vi "empty_string_values.vi"(11 "string refs":refnum<vi>[](array[refnum])) -> ()   [LabVIEW 2013]
panel:
  in  "Rino status control":T1={"Navigation controls"={"full path tree"=refnum, "folder content tree"=refnum, "next page"=refnum, "previous page"=refnum, "refresh file list"=refnum, "delete"=refnum, "page indicator string"=refnum}, "New Folder controls"={"next folder"=refnum, "name"="", "tags"="", "notes"="", "metadata array"=[]}, "Upload File controls"={"upoad file"=refnum, "name"="", "tags"="", "notes"="", "metadata array"=[], "Store data locally"=TRUE, "Store metadata locally"=FALSE, "Path Refnum"=refnum}, "Metadata management controls"={"get metadata"=refnum, "update metadata"=refnum, "name"=refnum, "tags"=refnum, "notes"=refnum, "metadata tree"=refnum}, "Status indicators"={"error"=refnum, "active item"=refnum, "last action"=refnum, "http header"=refnum, "http body"=refnum}, "Move file controls"={"source item"=refnum, "destination item"=refnum, "set source"=refnum, "set destination"=refnum, "move"=refnum}} {"Upload File controls"."metadata array"."Data type" items=["Numeric", "String", "1D array of strings", "1D array of doubles", "Data JSON string", "<null>"]; "New Folder controls"."metadata array"."Data type" items=["Numeric", "String", "1D array of strings", "1D array of doubles", "Data JSON string", "<null>"]}
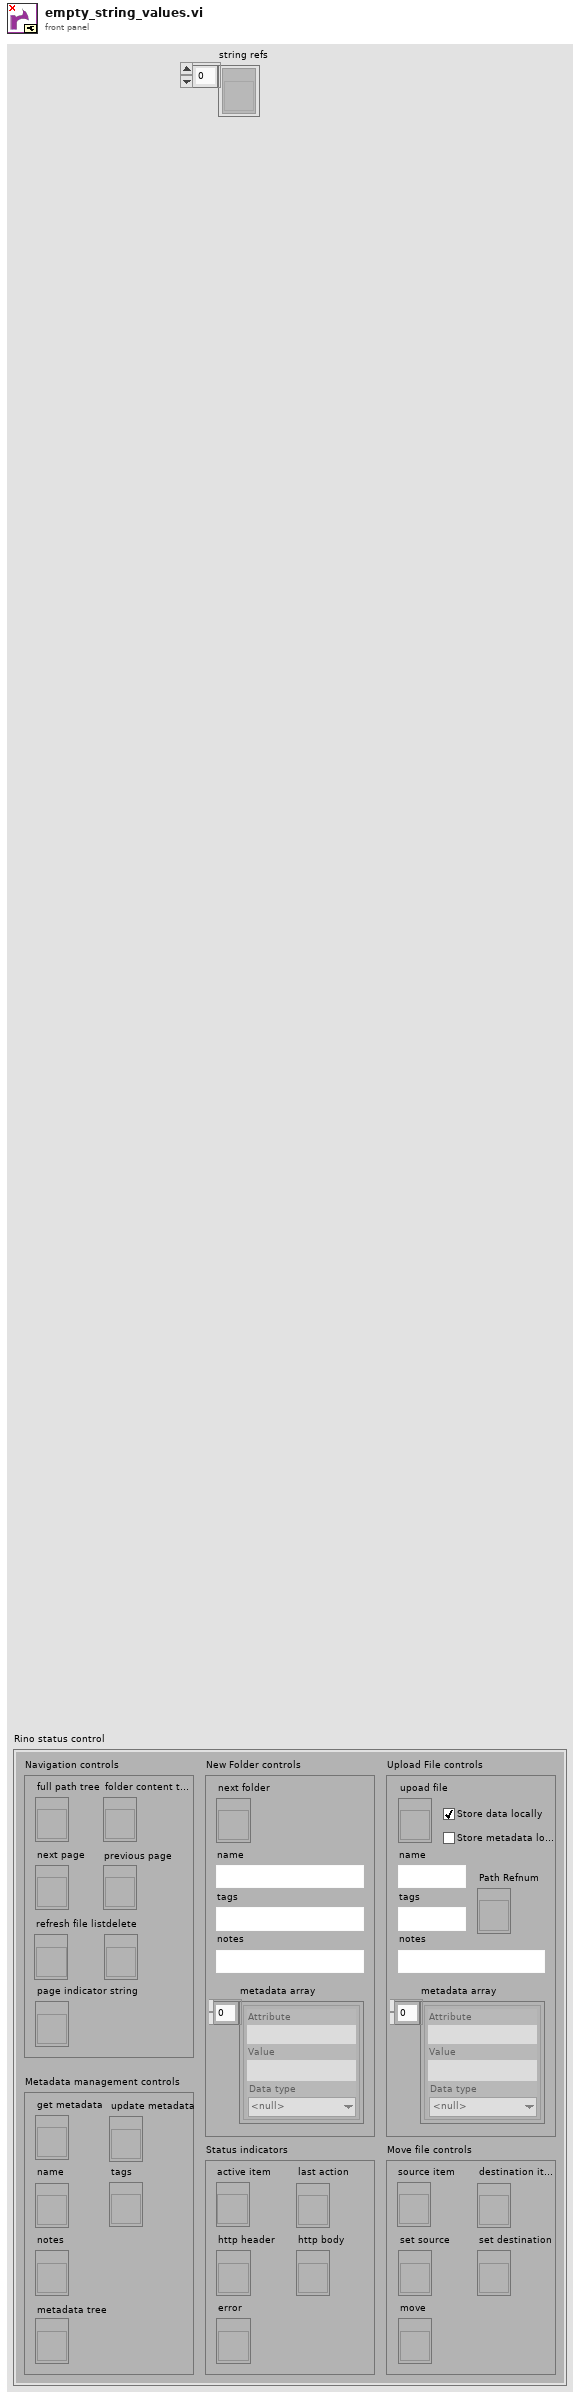
[diagram p1: front panel]
types:
  T1 = cluster{"Navigation controls":cluster{"full path tree":refnum<vi>, "folder content tree":refnum<vi>, "next page":refnum<vi>, "previous page":refnum<vi>, "refresh file list":refnum<vi>, "delete":refnum<vi>, "page indicator string":refnum<vi>}, "New Folder controls":cluster{"next folder":refnum<vi>, "name":string, "tags":string, "notes":string, "metadata array":cluster{"Attribute":string, "Value":string, "Data type":u16}[]}, "Upload File controls":cluster{"upoad file":refnum<vi>, "name":string, "tags":string, "notes":string, "metadata array":cluster{"Attribute":string, "Value":string, "Data type":u16}[], "Store data locally":bool, "Store metadata locally":bool, "Path Refnum":refnum<vi>}, "Metadata management controls":cluster{"get metadata":refnum<vi>, "update metadata":refnum<vi>, "name":refnum<vi>, "tags":refnum<vi>, "notes":refnum<vi>, "metadata tree":refnum<vi>}, "Status indicators":cluster{"error":refnum<vi>, "active item":refnum<vi>, "last action":refnum<vi>, "http header":refnum<vi>, "http body":refnum<vi>}, "Move file controls":cluster{"source item":refnum<vi>, "destination item":refnum<vi>, "set source":refnum<vi>, "set destination":refnum<vi>, "move":refnum<vi>}}
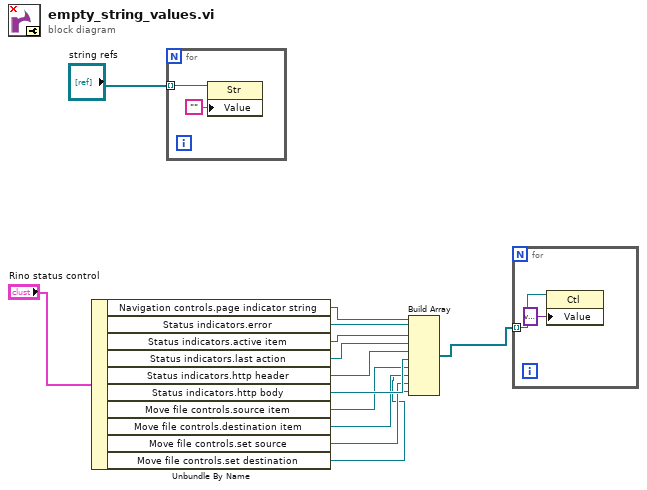
[diagram p0: block diagram]
diagram:
  n1 = Unbundle By Name("Rino status control") -> ("Navigation controls.page indicator string"=w11:refnum<vi>, "Status indicators.error"=w10:refnum<vi>, "Status indicators.active item"=w9:refnum<vi>, "Status indicators.last action"=w8:refnum<vi>, "Status indicators.http header"=w7:refnum<vi>, "Status indicators.http body"=w6:refnum<vi>, "Move file controls.source item"=w5:refnum<vi>, "Move file controls.destination item"=w4:refnum<vi>, "Move file controls.set source"=w3:refnum<vi>, "Move file controls.set destination"=w2:refnum<vi>)
  n2 = for {
    tunnel: "string refs" -> [w15] mode=indexing
    n3 = property class="Str"(reference=w15, "Value"="") -> ()  [unwired: 1 in, 2 out]
  }
  n4 = Build Array(w11, w10, w9, w8, w7, w6, w5, w4, w3, w2) -> (w1:refnum<vi>[])
  n5 = for {
    tunnel: w1 -> [w17] mode=indexing
    n6 = property class="Ctl"(reference=w17, "Value"=variant) -> ()  [unwired: 1 in, 2 out]
  }
